vi "Display.vi"(6 "include timestamp? (F)":bool, 7 "prefix (\"\")":string, 8 "error in (no error)":errorcluster, 9 "clear before next write (F)":bool, 11 "log text":string) -> (0 "error out":errorcluster)   [LabVIEW 2017, in "Debug Log.lvlib"]
doc: "Use this VI to log strings generated at various points in your program. Each time you call it, it appends <b>prefix</b> + <b>log text</b> to the displayed string, optionally including a timestamp. This VI opens on first call and remains open even after the program terminates.\n\nThis VI executes even if <b>error in</b> indicates an error."
uses:
  <vilib>/Utility/Debug Log/Debug Log.lvlib
panel:
  in  "Clear before next write":bool
  out "Log":string
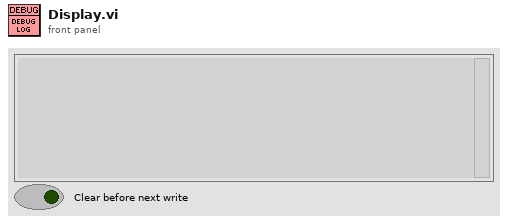
[diagram p1: front panel]
types:
  T1 = enum32{"Invalid", "Standard", "Closed", "Hidden", "Minimized", "Maximized"}
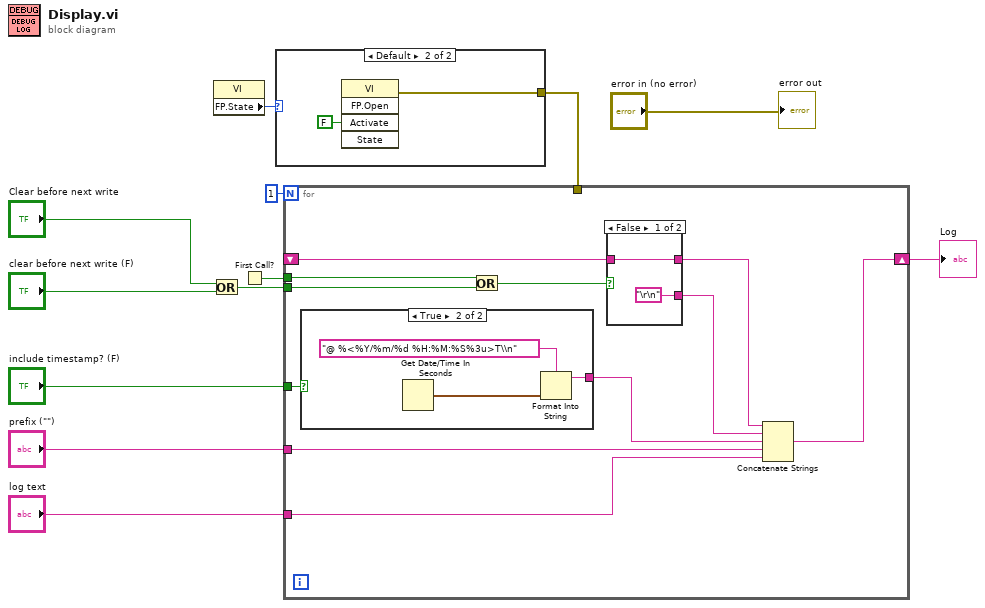
[diagram p0: block diagram]
diagram:
  n1 = Or(x="Clear before next write", y="clear before next write (F)") -> (x .or. y?=w1:bool)
  n2 = property class="VI"() -> ("FP.State"=w4:T1)  [unwired: 2 in, 2 out]
  n3 = First Call?() -> (First Call?: T/F=w5:bool)
  n4 = case shown="Default" w4 {
    tunnel: [_ w13] -> w8
    frame "Standard", "Minimized", "Maximized" {
    }
    frame Default {
      n5 = invoke class="VI" method="FP.Open"("Activate"=FALSE ("Activate?")) -> (error out=w13:errorcluster)  [unwired: 4 in, 4 out]
    }
  }
  n6 = for {
    N: 1 -> [_]
    shift-right: [w25] -> w7
    shift-left: _ -> [w23]
    tunnel: "log text" -> [w21]
    tunnel: w1 -> [w20]
    tunnel: "prefix (\"\")" -> [w18]
    tunnel: w8 -> [_]
    tunnel: "include timestamp? (F)" -> [w17]
    tunnel: w5 -> [w15]
    n7 = case shown="True" w17 {
      tunnel: [_ w28] -> w16
      frame False {
      }
      frame True {
        n8 = Get Date/Time In Seconds() -> (seconds since 1Jan1904=w27:timestamp)
        n9 = Format Into String(format string="@ %<%Y/%m/%d %H:%M:%S%3u>T\\n", w27) -> (resulting string=w28:string)  [unwired: 2 in, 1 out]
      }
    }
    n10 = Or(x=w15, y=w20) -> (x .or. y?=w22:bool)
    n11 = case shown="False" w22 {
      tunnel: [w30 _] -> w24
      tunnel: w23 -> [w30 _]
      tunnel: ["\r\n" _] -> w19
      frame False {
      }
      frame True {
      }
    }
    n12 = Concatenate Strings(w24, w19, w16, w18, w21) -> (w25:string)
  }
  "Log" <- w7
  "error out" <- "error in (no error)"
